vi "Difference Quotient (single).vi"(6 "Type":enum16{"y/x vs x", "x/y vs y"}(ring), 8 "error in (no error)":errorcluster, 9 "Interval Units (points)":enum16{"Points", "Data"}(ring), 10 "Window [h] (2)":dbl=2.0, 11 "XY-data":cluster{"X-array":dbl[], "Y-array":dbl[]}) -> (0 "error out":errorcluster, 2 "Difference Quotient":cluster{"X-array":dbl[], "Y-array":dbl[]} {"Y-array" format="%.2p"; "X-array" format="%.2p"}, 3 "XY-data out":cluster{"X-array":dbl[], "Y-array":dbl[]})   [LabVIEW 2019, in "xy_utilities.lvlib"]
doc: "Calculate the difference quotient (y[i-h/2]-y[i+h/s])/(x[i-h/2]-x[i+h/2]).\n\nWire data to the data input to determine the polymorphic instance to use or manually select the instance."
uses:
  xy_utilities.lvlib
  Swap X and Y (single).vi
  Reverse (single).vi
  Add XY (single).vi
  Divide float (single).vi
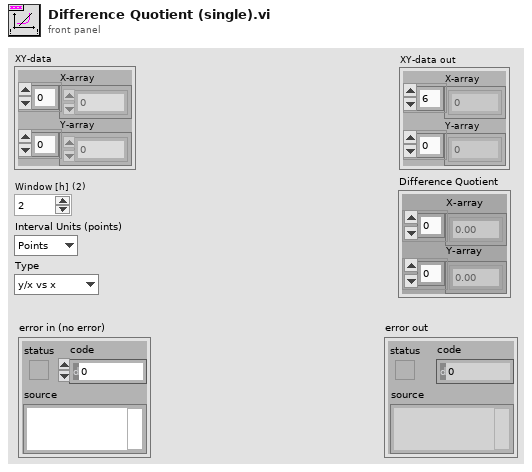
[diagram p1: front panel]
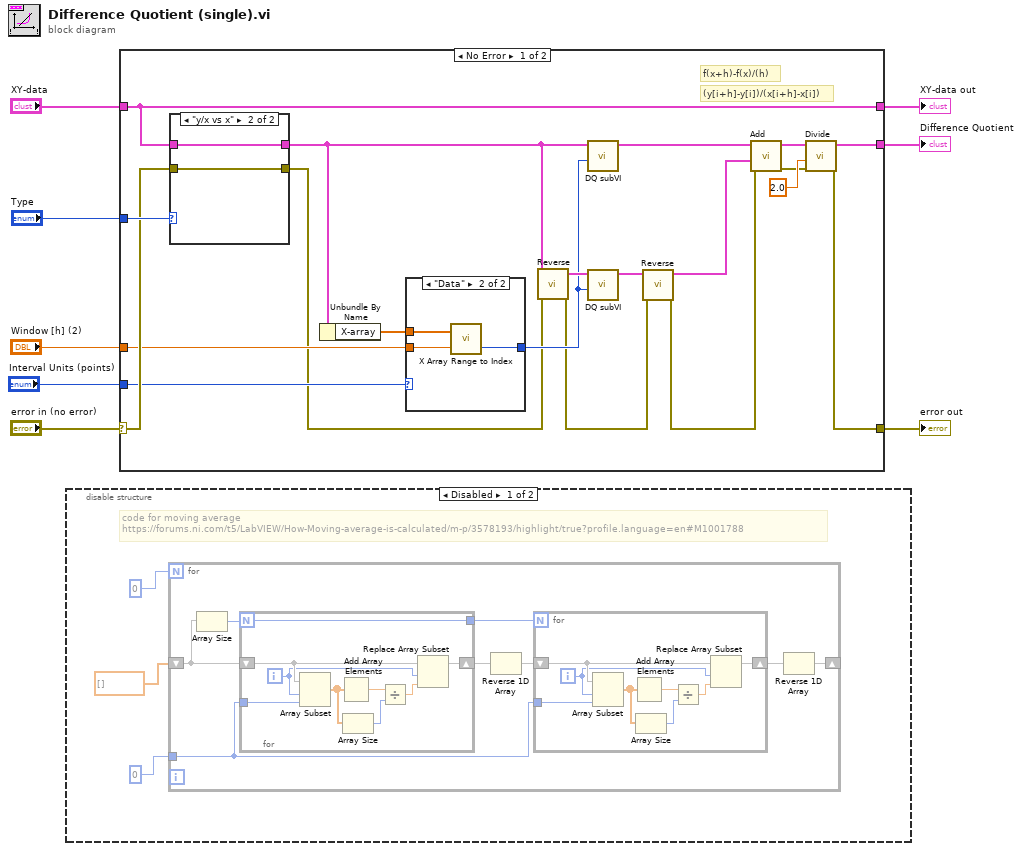
[diagram p0: block diagram]
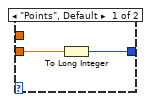
[diagram p3: hidden frame]
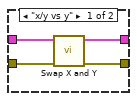
[diagram p4: hidden frame]
diagram:
  n1 = disable-structure shown="Disabled" {
    frame Disabled {
      # "code for moving average\nhttps://forums.ni.com/t5/LabVIEW/How-Moving-average-is-calculated/m-p/3578193/highlight/true?profile.language=en#M1001788"
      n2 = for {
        N: 0 ("iterations") -> [_]
        tunnel: 0 ("Window") -> [w15]
        shift-right: [w14] -> _
        shift-left: dbl[] [] ("Data In") -> [w19]
        n3 = Array Size(array=w19) -> (size(s)=w13:i32)
        n4 = for {
          N: w13 -> [w28]
          shift-right: [w32] -> w18
          shift-left: w19 -> [w35]
          tunnel: w15 -> [w31]
          tunnel: [w28] -> w12
          i -> [w34]
          n5 = Array Subset(array=w35, index=w34, length=w31) -> (w30:dbl[])
          n6 = Add Array Elements(numeric array=w30) -> (sum=w36:dbl)
          n7 = Array Size(array=w30) -> (size(s)=w29:i32)
          n8 = Divide(x=w36, y=w29) -> (x/y=w33:dbl)
          n9 = Replace Array Subset(array=w35, new element=w33, index=w34) -> (w32:dbl[])
        }
        n10 = Reverse 1D Array(array=w18) -> (reversed array=w17:dbl[])
        n11 = for {
          N: w12 -> [_]
          shift-right: [w23] -> w16
          shift-left: w17 -> [w26]
          tunnel: w15 -> [w22]
          i -> [w25]
          n12 = Array Subset(array=w26, index=w25, length=w22) -> (w21:dbl[])
          n13 = Add Array Elements(numeric array=w21) -> (sum=w27:dbl)
          n14 = Array Size(array=w21) -> (size(s)=w20:i32)
          n15 = Divide(x=w27, y=w20) -> (x/y=w24:dbl)
          n16 = Replace Array Subset(array=w26, new element=w24, index=w25) -> (w23:dbl[])
        }
        n17 = Reverse 1D Array(array=w16) -> (reversed array=w14:dbl[])
      }
    }
    frame Enabled {
    }
  }
  n18 = case shown="No Error" "error in (no error)" {
    selector: "error in (no error)" -> [w55 w69]
    tunnel: [w39 w69] -> w7
    tunnel: "XY-data" -> [w54 w68]
    tunnel: [w44 _] -> w5
    tunnel: "Type" -> [w56 _]
    tunnel: [w54 w68] -> w3
    tunnel: "Window [h] (2)" -> [w53 _]
    tunnel: "Interval Units (points)" -> [w52 _]
    frame No Error {
      # "(y[i+h]-y[i])/(x[i+h]-x[i])"
      # "f(x+h)-f(x)/(h)"
      n19 = case shown="\"y/x vs x\"" w56 {
        tunnel: w54 -> [w65 w67]
        tunnel: [w64 w67] -> w50
        tunnel: [w63 w66] -> w43
        tunnel: w55 -> [w62 w66]
        frame "x/y vs y" {
          n20 = call-poly "Swap X and Y.vi"("error in (no error)"=w62, "XY-data"=w65) -> ("error out"=w63:errorcluster, "XY-data out"=w64:cluster{"X-array":dbl[], "Y-array":dbl[]})  [unwired: 8 in]
        }
        frame "y/x vs x" {
        }
      }
      n21 = Unbundle By Name(w50) -> ("X-array"=w51:dbl[])
      n22 = case shown="\"Data\"" w52 {
        tunnel: w51 -> [_ w61]
        tunnel: w53 -> [w58 w60]
        tunnel: [w57 w59] -> w48
        frame "Points", Default {
          n23 = To Long Integer(number=w58) -> (32bit integer=w57:i32)
        }
        frame "Data" {
          n24 = call "X Array Range to Index.vi"("X Range"=w60, "X-array"=w61) -> ("X Range (index)"=w59:i32)  [unwired: 1 in]
        }
      }
      n25 = call-poly "Reverse.vi"("error in (no error)"=w43, "XY-data"=w50) -> ("error out"=w42:errorcluster, "Reversed XY-data out"=w49:cluster{"X-array":dbl[], "Y-array":dbl[]})  [unwired: 8 in]
      n26 = call "DQ subVI.vi"("window (h)"=w48, "XY-data"=w50) -> ("XY-data out"=w38:cluster{"X-array":dbl[], "Y-array":dbl[]})  [unwired: 9 in]
      n27 = call "DQ subVI.vi"("window (h)"=w48, "XY-data"=w49) -> ("XY-data out"=w47:cluster{"X-array":dbl[], "Y-array":dbl[]})  [unwired: 9 in]
      n28 = call-poly "Reverse.vi"("error in (no error)"=w42, "XY-data"=w47) -> ("error out"=w40:errorcluster, "Reversed XY-data out"=w37:cluster{"X-array":dbl[], "Y-array":dbl[]})  [unwired: 8 in]
      n29 = call-poly "Add.vi"("error in (no error)"=w40, "y"=w37, "XY-data"=w38) -> ("error out"=w41:errorcluster, "XY-data out"=w46:cluster{"X-array":dbl[], "Y-array":dbl[]})  [unwired: 7 in]
      n30 = call-poly "Divide.vi"("error in (no error)"=w41, "y (1)"=2.0, "XY-data"=w46) -> ("error out"=w39:errorcluster, "XY-data out"=w44:cluster{"X-array":dbl[], "Y-array":dbl[]})  [unwired: 7 in]
    }
    frame Error {
    }
  }
  "error out" <- w7
  "Difference Quotient" <- w5
  "XY-data out" <- w3
